vi "Setup TestRunner Folder.vi"(5 "Interactive (T)":bool=TRUE, 6 "Inspect Recursively (T)":bool=TRUE, 7 "Verbose (F)":bool, 8 "error in (no error)":errorcluster, 9 "Test Report":refnum<class "Test Report.lvclass">, 10 "Directory to search":path, 11 "Test Runner.Folder":refnum<class "Test Runner.Folder.lvclass">) -> (0 "error out":errorcluster, 3 "Test Runner.Folder out":refnum<class "Test Runner.Folder.lvclass">)   [LabVIEW 2013, in "Caraya.lvlib" / "Test Runner.Folder.lvclass"]
uses:
  Test Runner.Folder/Test Runner.Folder.lvclass
  Test Report/Test Report.lvclass
  Test Runner.lvclass/Test Runner.ctl
  Test Runner.Folder/Test Runner.Folder.lvclass/Test Runner.Folder.ctl
  Test Runner.lvclass
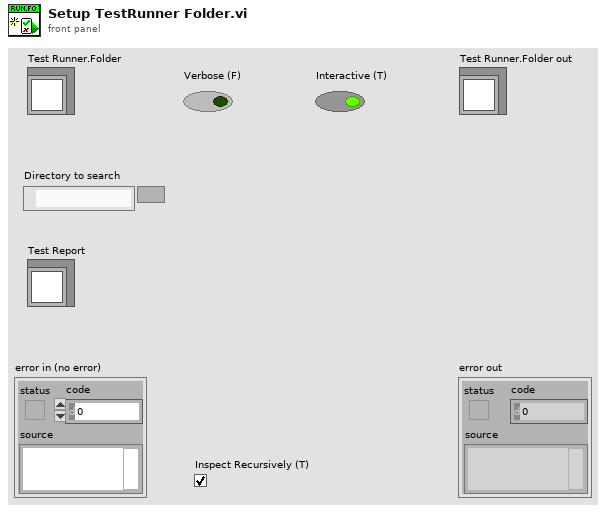
[diagram p1: front panel]
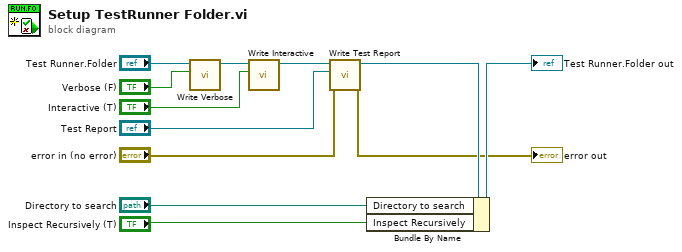
[diagram p0: block diagram]
diagram:
  n1 = call "Write Verbose.vi"("Verbose"="Verbose (F)", "Test Runner in"="Test Runner.Folder") -> ("Test Runner out"=w5:refnum<class "Test Runner.Folder.lvclass">)  [unwired: 9 in]
  n2 = call "Write Interactive.vi"("Interactive"="Interactive (T)", "Test Runner in"=w5) -> ("Test Runner out"=w4:refnum<class "Test Runner.Folder.lvclass">)  [unwired: 9 in]
  n3 = call-dynamic "Write Test Report.vi"("error in (no error)"="error in (no error)", "Test Report"="Test Report", "Test Runner in"=w4) -> ("error out"=→"error out":errorcluster, "Test Runner out"=w10:refnum<class "Test Runner.Folder.lvclass">)  [unwired: 7 in]
  n4 = Bundle By Name(cluster=w10, "Directory to search"="Directory to search", "Inspect Recursively"="Inspect Recursively (T)") -> (→"Test Runner.Folder out":refnum<class "Test Runner.Folder.lvclass">)
